vi "Instrumentation.vi"() -> ()   [LabVIEW 2015]
panel:
  out "Slide 6":u8(slide) scale=0.0..100.0
  out "Slide 5":u8(slide) scale=0.0..100.0
  out "Slide 4":u8(slide) scale=0.0..100.0
  out "Slide 3":u8(slide) scale=0.0..100.0
  out "Slide 2":u8(slide) scale=0.0..100.0
  out "Slide":u8(slide) scale=0.0..100.0
  out "Numeric 3":dbl
  out "Numeric 2":dbl
  out "Numeric":dbl
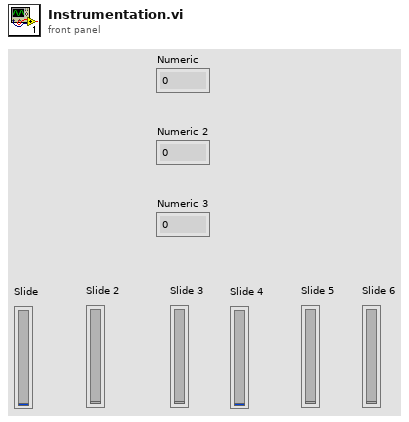
[diagram p1: front panel]
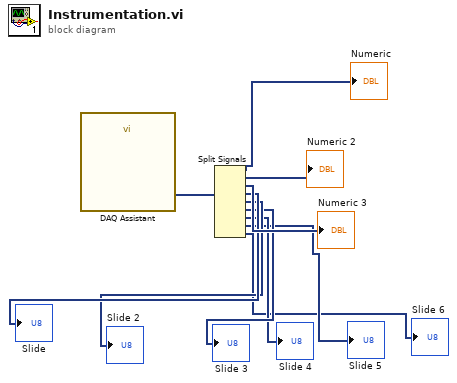
[diagram p0: block diagram]
diagram:
  n1 = call "DAQ Assistant"() -> ("data"=w10:dynamicdata)  [unwired: 17 in, 2 out]
  n2 = Split Signals(w10) -> (→"Numeric":dynamicdata, →"Numeric 2":dynamicdata, →"Numeric 3":dynamicdata, →"Slide":dynamicdata, →"Slide 2":dynamicdata, →"Slide 3":dynamicdata, →"Slide 4":dynamicdata, →"Slide 5":dynamicdata, →"Slide 6":dynamicdata)  [unwired: 9 in]
